vi "Actualizar Estatus.vi"(8 "error in (no error)":errorcluster, 9 "ACTUALIZA TABLA":bool, 10 "ESTATUS":string, 11 "UI Actor in":refnum<class "UI Actor.lvclass">) -> (0 "error out":errorcluster, 3 "UI Actor out":refnum<class "UI Actor.lvclass">)   [LabVIEW 2019, in "UI Actor.lvlib" / "UI Actor.lvclass"]
uses:
  UI Actor.lvclass
  UI Actor.lvclass/UI Actor.ctl
  MENSAJES Messages/Actualiza Mensaje Msg/Actualiza Mensaje Msg.lvclass/Actualiza Mensaje Msg.ctl
  <vilib>/ActorFramework/Message Enqueuer/Message Enqueuer.lvclass/Message Enqueuer.ctl
  CAFE ACTOR Messages/Actualiza Tabla Msg/Actualiza Tabla Msg.lvclass/Actualiza Tabla Msg.ctl
  REFRESCOS Y PAPAS ACTOR Messages/Actualiza Tabla Msg/Actualiza Tabla Msg.lvclass/Actualiza Tabla Msg.ctl
  <vilib>/ActorFramework/Message Enqueuer/Enqueue.vi
  MENSAJES Messages/Actualiza Mensaje Msg/Actualiza Mensaje Msg.lvclass
  C:/Program Files (x86)/National Instruments/LabVIEW 2019/vi.lib/ActorFramework/Message/Message.lvclass
  CAFE ACTOR Messages/Actualiza Tabla Msg/Actualiza Tabla Msg.lvclass
  REFRESCOS Y PAPAS ACTOR Messages/Actualiza Tabla Msg/Actualiza Tabla Msg.lvclass
  <vilib>/ActorFramework/Message Priority Queue/Priority Enqueue.vi
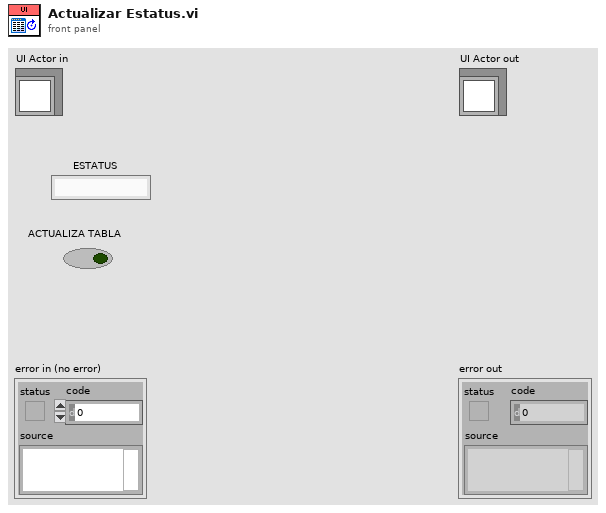
[diagram p1: front panel]
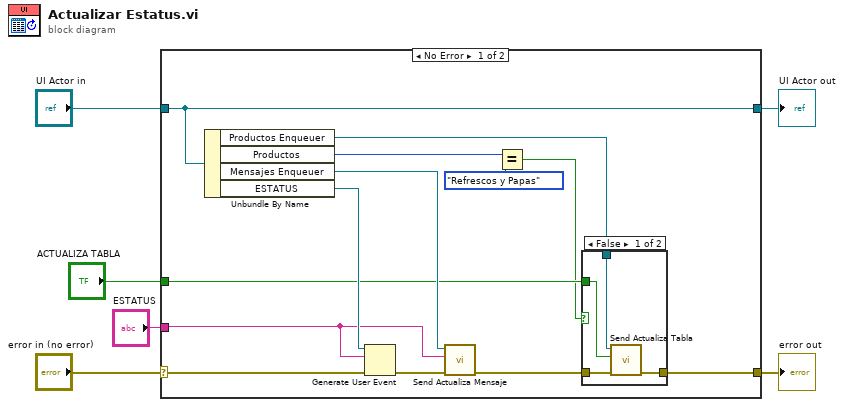
[diagram p0: block diagram]
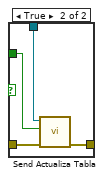
[diagram p2: hidden frame]
diagram:
  n1 = case shown="No Error" "error in (no error)" {
    selector: "error in (no error)" -> [w18 w29]
    tunnel: [w12 w29] -> w5
    tunnel: [w19 w28] -> w3
    tunnel: "UI Actor in" -> [w19 w28]
    tunnel: "ESTATUS" -> [w14 _]
    tunnel: "ACTUALIZA TABLA" -> [w11 _]
    frame No Error {
      n2 = Unbundle By Name(w19) -> ("Productos Enqueuer"=w10:refnum<class "Message Enqueuer.lvclass">, "Productos"=w9:enum16{"Refrescos y Papas", "Cafe"}, "Mensajes Enqueuer"=w15:refnum<class "Message Enqueuer.lvclass">, "ESTATUS"=w17:refnum<user-event>)
      n3 = Generate User Event(user event=w17, event data cluster=w14, error in=w18) -> (error out=w16:errorcluster)  [unwired: 1 in, 1 out]
      n4 = call "Send Actualiza Mensaje.vi"("error in (no error)"=w16, "Mensaje Status"=w14, "Message Enqueuer"=w15) -> ("error out"=w13:errorcluster)  [unwired: 7 in, 1 out]
      n5 = Equal?(x=w9, y=enum16{"Refrescos y Papas", "Cafe"}."Refrescos y Papas") -> (x = y?=w7:bool)
      n6 = case shown="False" w7 {
        tunnel: w13 -> [w23 w27]
        tunnel: [w22 w26] -> w12
        tunnel: w11 -> [w20 w25]
        tunnel: w10 -> [w21 w24]
        frame False {
          n7 = call "Send Actualiza Tabla.vi"("error in (no error)"=w23, "ACTUALIZA TABLA"=w20, "Message Enqueuer"=w21) -> ("error out"=w22:errorcluster)  [unwired: 7 in, 1 out]
        }
        frame True {
          n8 = call "Send Actualiza Tabla.vi"("error in (no error)"=w27, "ACTUALIZA TABLA"=w25, "Message Enqueuer"=w24) -> ("error out"=w26:errorcluster)  [unwired: 7 in, 1 out]
        }
      }
    }
    frame Error {
    }
  }
  "error out" <- w5
  "UI Actor out" <- w3
